vi "Data Format_old.vi"() -> (0 "title":string[](array[string]), 1 "title_beforedata":string[](array[string])=["Date", "Time", "Test_Time", "Station_Name", "Station_ID", "Variant", "Cavity_ID", "Operator_ID", "Serial_Number", "MES_DDM_SN", "Attempt_Time", "ETS_No", "MES", "SKU", "Plate_Diameter", "Overall_Result", "Error_Code", "Error_Description", "Run_Mode"], 3 "数组":string[][](array[string]))   [LabVIEW 2017]
panel:
  out "Table":string[][](array[string])
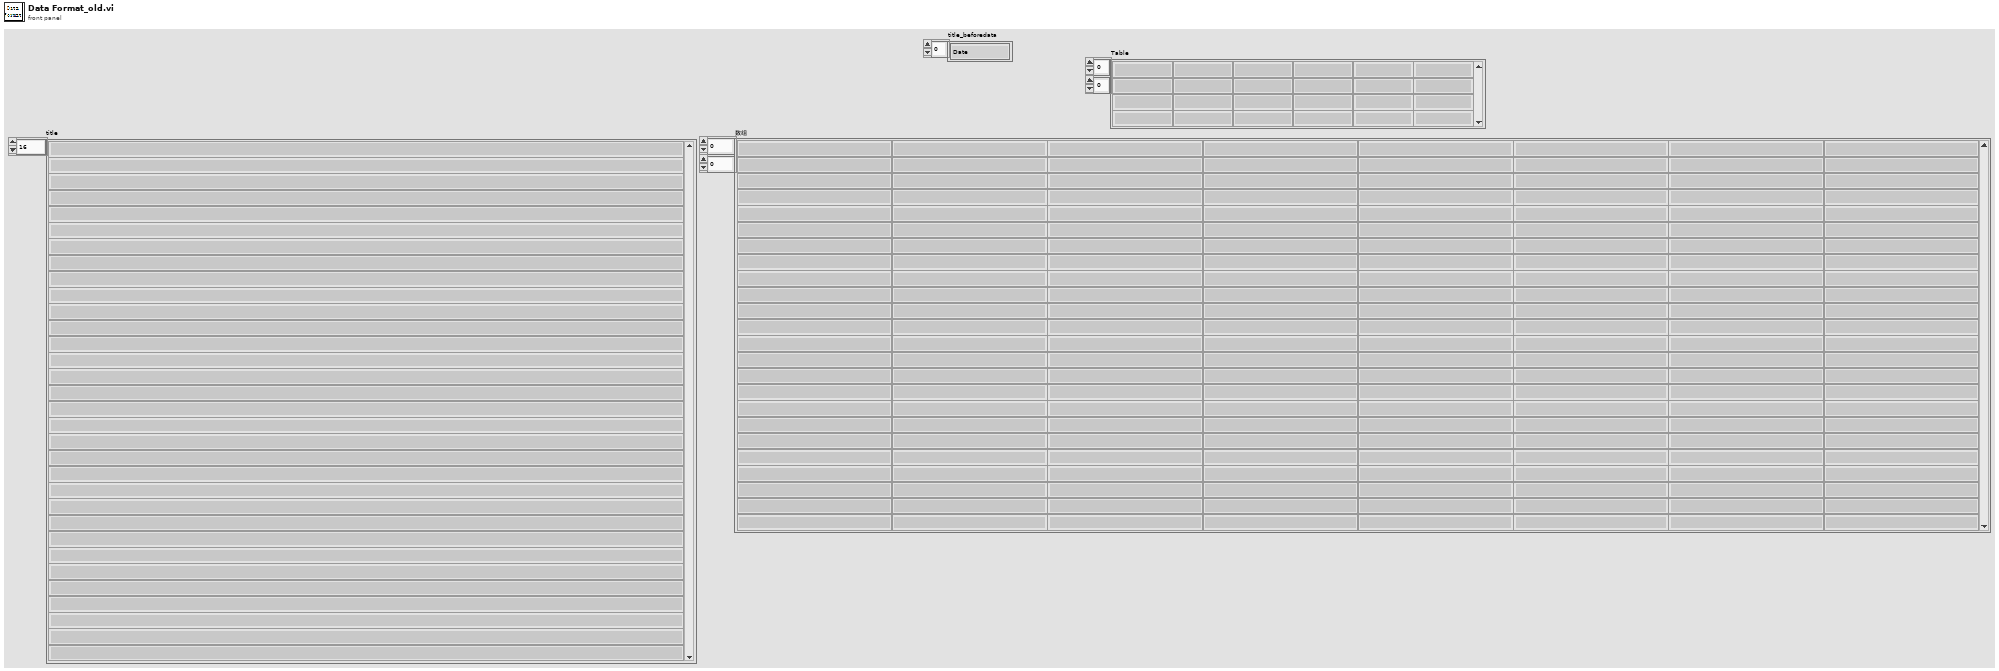
[diagram p1: front panel]
types:
  T1 = typedef "HD Config.ctl" = cluster{" PC":cluster{"PC Address":u8[], "PC Port":i32}, "FCO":cluster{"COM":refnum<visa-resource-name>, "Baudrate":u32}, "DC Power ":cluster{"COM":refnum<visa-resource-name>, "Baudrate":u32}, "PW3336":cluster{"COM":refnum<visa-resource-name>, "Baudrate":u32}, "Lefoo":cluster{"COM":refnum<visa-resource-name>, "Baudrate":u32}, "Tempt&Hum":cluster{"COM":refnum<visa-resource-name>, "Baudrate":u32}, "DIPC":cluster{"COM":refnum<visa-resource-name>}, "Daemon":cluster{"IP Address":string, "Port":u16, "Retry":u16}, "Motor":cluster{"COM":refnum<visa-resource-name>, "Baudrate":u32}, "Fail_resume_mode":bool, "GRR":bool}
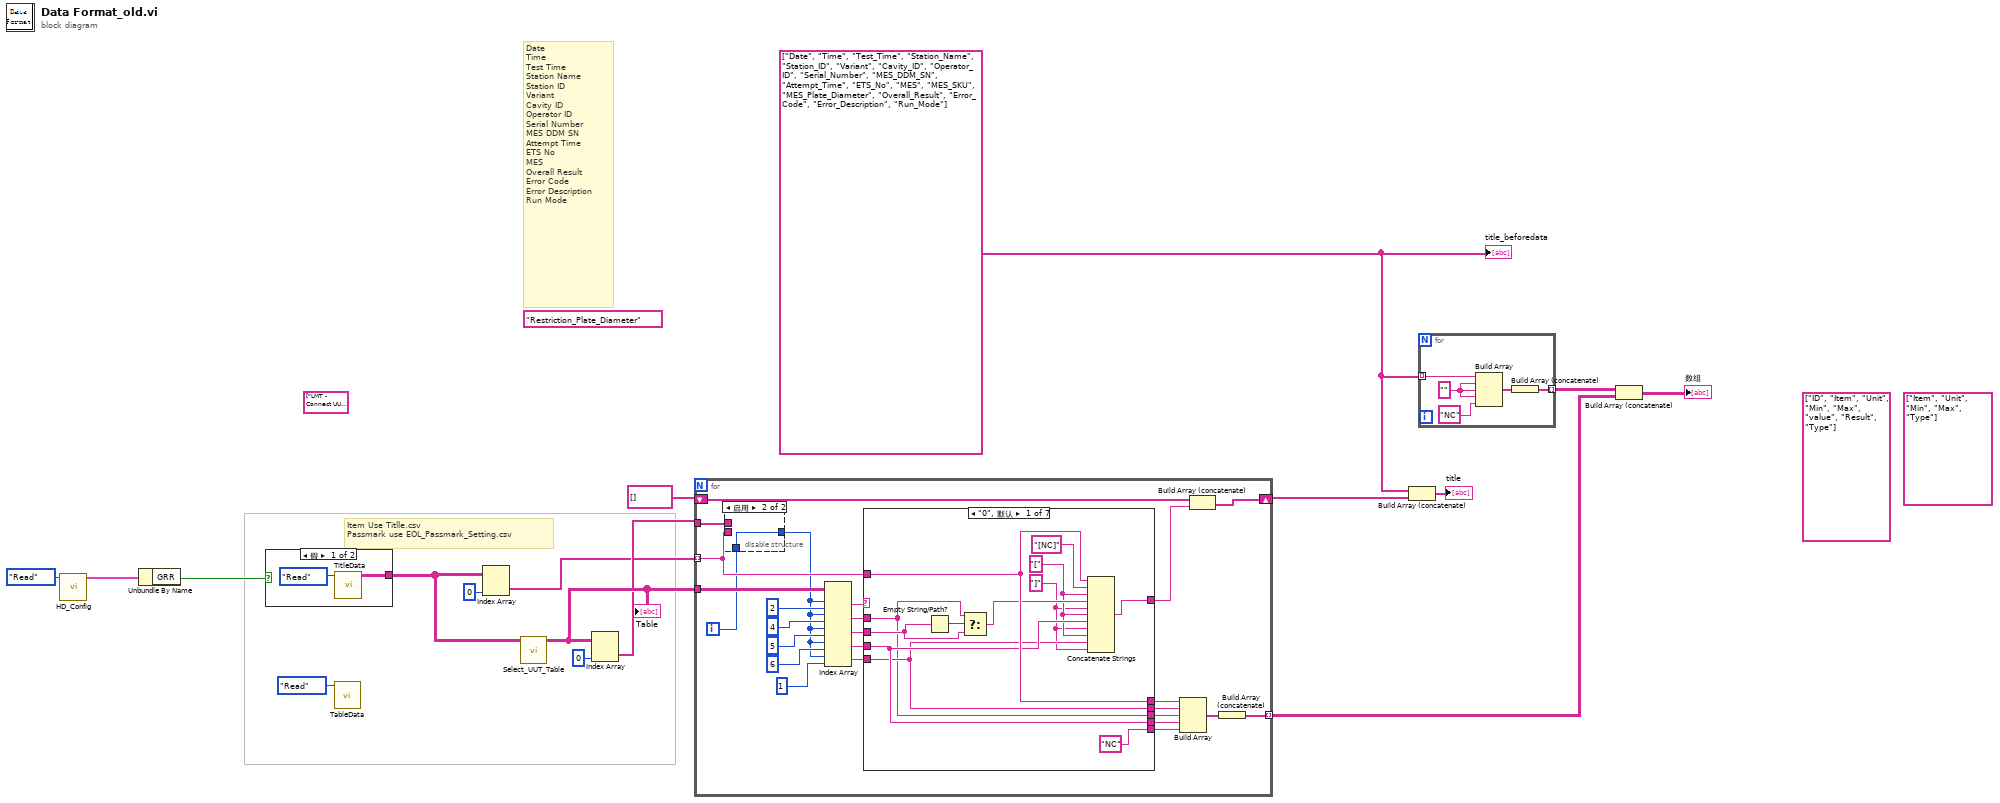
[diagram p0: block diagram]
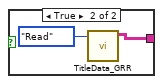
[diagram p2: hidden frame]
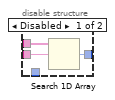
[diagram p3: hidden frame]
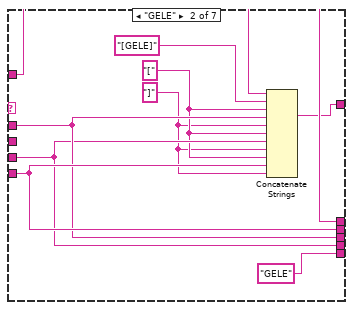
[diagram p4: hidden frame]
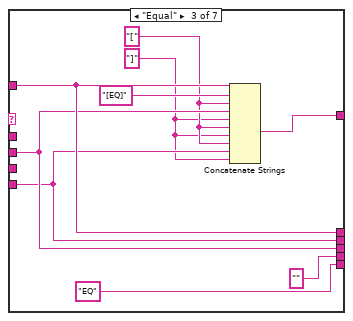
[diagram p5: hidden frame]
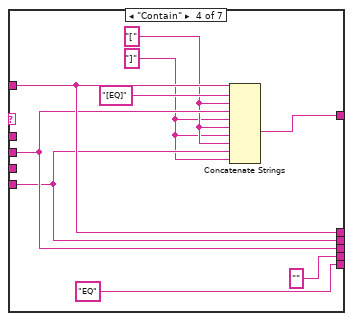
[diagram p6: hidden frame]
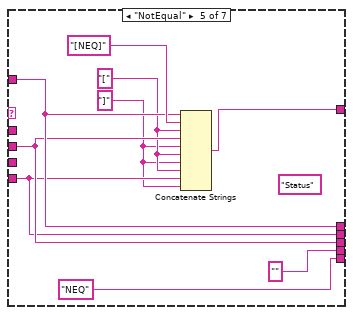
[diagram p7: hidden frame]
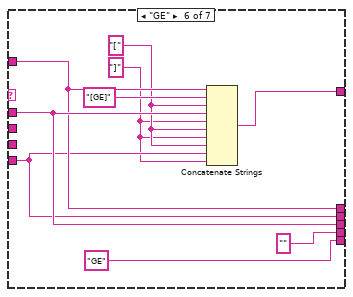
[diagram p8: hidden frame]
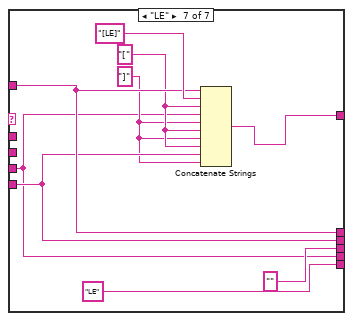
[diagram p9: hidden frame]
diagram:
  (unwired) "Restriction_Plate_Diameter"
  (unwired) string[] ["ID", "Item", "Unit", "Min", "Max", "value", "Result", "Type"] ("列首字符串[]")
  (unwired) string[] ["LMT - Connect UUT (con COM)", "LMT - Software Version (rrel)", "LMT - Write SKU file (wskuc)", "LMT - SKU file name", "LMT Connect UUT - Error Log", "5.3.2.1 Connect UUT DDM", "Connect UUT DDM - Error Log", "5.3.2.8 Read DDM EOL Timestamp", "5.3.2.8 Read DDM EOL Timestamp - Mode", "5.3.2.8 Read DDM EOL Timestamp - Timestamp", "5.3.2.8 Read DDM EOL Timestamp - Rig ID", "5.3.2.8 Read DDM EOL Timestamp - Passmark ID", "5.3.2.8 Read DDM EOL Timestamp - Passmark Rev", "Read DDM EOL Timestamp - Error Log", "5.3.2.2 Read DDM SW Version before flashing", "5.3.2.2 Software Version before flashing", "Read DDM SW Version before flashing - Error Log", "5.3.2.7 Read Hardware Serial", "Read Hardware Serial - Error Log", "Read DDM SN from UUT", "UUT DDM SN", "Compare Length", "Compare DDM SN with MES SN", "Check DDM SN - Error Log", "5.3.6.2.2 Backup File Data - CAL", "5.3.6.2.2 Backup Data Response - CAL", "5.3.2.3 Flash Firmware Version", "5.3.2.4 Wait Timeout", "5.3.2.5 Check SW Version", "5.3.2.5 Flashing firmware file name", "Flash Firmware Version - Error Log", "5.3.2a.1 Disconnect UUT", "Disconnect UUT - Error Log", "5.3.2a.3 Connect UUT UI", "Connect UUT UI - Error Log", "5.3.2a.4 Flash Firmware Version", "5.3.2a.4 Wait Timeout", "5.3.2a.4 Check SW Version", "5.3.2a.5 Flashing firmware file name", "Flash Firmware Version - Error Log", "5.3.2.6 Read DDM SW Version after flashing", "5.3.2.6 Check DDM SW Version after flashing", "Read DDM SW Version after flashing - Error Log", "5.3.2.10 Set SKU Config Status", "5.3.2.10 Set SKU Config", "5.3.2.10 Set SKU Config File Name", "Set SKU Config - Error Log", "5.3.2.10 Ready Status", "Ready Status - Error Log", "5.3.2.12 Set Device Mode to EOL", "5.3.2.12 DDM EOL mode", "Set Device Mode - Error Log", "5.3.4.34 Wait 1s", "5.3.2.13 DDM Parameter - Voltage", "5.3.2.13 DDM Parameter - Current", "5.3.2.13 DDM Parameter - Power", "5.3.2.13 DDM Parameter - Speed", "5.3.2.13 DDM Parameter - Pressure", "5.3.2.14 Tester Parameter - Voltage", "5.3.2.14 Tester Parameter - Current", "5.3.2.14 Tester Parameter - Power", "5.3.2.14 Tester Parameter - Ambient Pressure", "5.3.2.14 Tester Parameter - Ambient Temperature", "5.3.2.14 Tester Parameter - Pressure Box", "5.3.2.14 Tester Parameter - Reference Ambient Pressure", "5.3.2.15 Calculated Parameter - DDM Pressure Corrected", "5.3.2.15 Calculated Parameter - DDM Real Power", "5.3.2.15 Calculated Parameter - Delta V", "Get and Check Parameter - Error Log", "5.3.3.0 Read BEMF ambient temperature", "5.3.3.0 Calibration Result - eol_cold_bemf_temp", "Read BEMF ambient temperature - Error Log", "5.3.3.0 Set ambient temp to DDM", "5.3.3.0 DDM Ambient Temp", "Set ambient temp to DDM - Error Log", "5.3.4.2 Restriction Plate Diameter", "5.3.4.2 BEMF CAL - Put 13mm Restriction Plate", "Put Restriction Plate - Error Log", "5.3.3.1 Set - Calibrate BEMF both", "5.3.3.1 Get - Calibrate BEMF LSI", "5.3.3.2 Get - Calibration Result - eol_bemf_mp_cold_coef_a", "5.3.3.2 Get - Calibration Result - eol_bemf_mp_cold_coef_b", "5.3.3.2 Get - Calibration Result - eol_bemf_mp_cold_coef_c", "5.3.3.2 Get - Calibration Result - eol_bemf_lsi_cold_ref_coeffs", "5.3.3.2 Get - Calibration Result - eol_bemf_lsi_speed", "5.3.3.2 Get - Calibration Result - eol_bemf_lsi_integral_0", "5.3.3.2 Get - Calibration Result - eol_bemf_lsi_integral_1", "5.3.3.2 Get - Calibration Result - eol_bemf_lsi_integral_2", "5.3.3.2 Get - Calibration Result - eol_cold_bemf", "5.3.3.2 Get - Calibration Result - eol_cold_bemf_fisf", "Get - Calibrate BEMF LSI - Error Log", "5.3.3.3 Finalise Calibration", "5.3.3.4 Wait 1 sec", "Finalise Calibration - Error Log", "5.3.3.1 Get - Calibrate BEMF LSI", "5.3.3.2 Get - Calibration Result - eol_cold_bemf", "5.3.3.2 Get - Calibration Result - eol_cold_bemf_fisf", "5.3.3.2 Compare -Calibration Result - eol_cold_bemf", "5.3.3.2 Compare -Calibration Result - eol_cold_bemf_fisf", "Get & Compare - Calibrate BEMF LSI - Error Log", "5.3.3.3 Reset Power Tune", "5.3.3.4 Reset Power Tune Value", "Reset Power Tune - Error Log", "5.3.3.3 Reset BEMF FISF Calibration", "5.3.3.4 Reset BEMF FISF Calibration Value", "Reset BEMF FISF Calibration - Error Log", "5.3.4.2 ECO - Put 13mm Restriction Plate", "5.3.4.2 Restriction Plate Diameter", "Put Restriction Plate - Error Log", "5.3.4.5 ECO - Motor ON", "5.3.4.5 ECO - Motor ON Mode", "ECO - Motor ON - Error Log", "5.3.4.6 ECO - Motor Speed Stabilisation", "5.3.4.6 ECO - Stabilisation Time", "ECO - Motor Speed Stabilisation - Error Log", "5.3.4.7 ECO - DDM Parameter - Voltage", "5.3.4.7 ECO - DDM Parameter - Current", "5.3.4.7 ECO - DDM Parameter - Power", "5.3.4.7 ECO - DDM Parameter - Measured Power", "5.3.4.7 ECO - DDM Parameter - Speed", "5.3.4.7 ECO - DDM Parameter - Pressure", "5.3.4.7 ECO - DDM Parameter - lsi magnet temp", "5.3.4.7 ECO - DDM Parameter - fisf magnet temp", "5.3.4.7 ECO - DDM Parameter - iir magnet temp", "5.3.4.8 ECO - Tester Parameter - Voltage", "5.3.4.8 ECO - Tester Parameter - Current", "5.3.4.8 ECO - Tester Parameter - Power", "5.3.4.8 ECO - Tester Parameter - Ambient Pressure", "5.3.4.8 ECO - Tester Parameter - Ambient Temperature", "5.3.4.8 ECO - Tester Parameter - Ambient Humidity", "5.3.4.8 ECO - Tester Parameter - Pressure Box", "5.3.4.8 ECO - Tester Parameter - Reference Ambient Pressure", "5.3.4.9 ECO - Calculated Parameter - DDM Pressure Corrected", "5.3.4.9 ECO - Calculated Parameter - DDM Real Power", "5.3.4.9 ECO - Calculated Parameter - Delta V", "5.3.4.9 ECO - Calculated Parameter - Flowrate", "5.3.4.9 ECO - Calculated Parameter - Airwatt", "5.3.4.9 ECO - Formula", "ECO - Get and Check Parameter - Error Log", "PT ECO - Power Tune Mode Status", "PT ECO - Power Tune Set Delta Power Tune", "PT ECO - Power Tune Index", "PT ECO - Power Tune Delta_P", "PT ECO - Power Tune Motor ON Status", "PT ECO - Power Tune Motor ON Mode", "PT ECO - Power Tune Stabilisation Time Status", "PT ECO - Power Tune Stabilisation Delay Time", "PT ECO - DDM Parameter - Voltage", "PT ECO - DDM Parameter - Current", "PT ECO - DDM Parameter - Power", "PT ECO - DDM Parameter - Measured Power", "PT ECO - DDM Parameter - Speed", "PT ECO - DDM Parameter - Pressure", "PT ECO - DDM Parameter - lsi magnet temp", "PT ECO - DDM Parameter - fisf magnet temp", "PT ECO - DDM Parameter - iir magnet temp", "PT ECO - Tester Parameter - Voltage", "PT ECO - Tester Parameter - Current", "PT ECO - Tester Parameter - Power", "PT ECO - Tester Parameter - Ambient Pressure", "PT ECO - Tester Parameter - Ambient Temperature", "PT ECO - Tester Parameter - Ambient Humidity", "PT ECO - Tester Parameter - Pressure Box", "PT ECO - Tester Parameter - Reference Ambient Pressure", "PT ECO - Calculated Parameter - DDM Pressure Corrected", "PT ECO - Calculated Parameter - DDM Real Power", "PT ECO - Calculated Parameter - Delta V", "PT ECO - Calculated Parameter - Flowrate", "PT ECO - Calculated Parameter - Airwatt", "PT ECO - Formula", "PT ECO - Get and Check Parameter - Error Log", "5.3.4.2 BOOST - Put 13mm Restriction Plate", "5.3.4.2 Restriction Plate Diameter", "Put Restriction Plate - Error Log", "5.3.4.5 BOOST - Motor ON", "5.3.4.5 BOOST - Motor ON Mode", "BOOST - Motor ON - Error Log", "5.3.4.6 BOOST - Motor Speed Stabilisation", "5.3.4.6 BOOST - Stabilisation Time", "5.3.4.7 BOOST - DDM Parameter - Voltage", "5.3.4.7 BOOST - DDM Parameter - Current", "5.3.4.7 BOOST - DDM Parameter - Power", "5.3.4.7 BOOST - DDM Parameter - Measured Power", "5.3.4.7 BOOST - DDM Parameter - Speed", "5.3.4.7 BOOST - DDM Parameter - Pressure", "5.3.4.7 BOOST - DDM Parameter - lsi magnet temp", "5.3.4.7 BOOST - DDM Parameter - fisf magnet temp", "5.3.4.7 BOOST - DDM Parameter - iir magnet temp", "5.3.4.8 BOOST - Tester Parameter - Voltage", "5.3.4.8 BOOST - Tester Parameter - Current", "5.3.4.8 BOOST - Tester Parameter - Power", "5.3.4.8 BOOST - Tester Parameter - Ambient Pressure", "5.3.4.8 BOOST - Tester Parameter - Ambient Temperature", "5.3.4.8 BOOST - Tester Parameter - Ambient Humidity", "5.3.4.8 BOOST - Tester Parameter - Pressure Box", "5.3.4.8 BOOST - Tester Parameter - Reference Ambient Pressure", "5.3.4.9 BOOST - Calculated Parameter - DDM Pressure Corrected", "5.3.4.9 BOOST - Calculated Parameter - DDM Real Power", "5.3.4.9 BOOST - Calculated Parameter - Delta V", "5.3.4.9 BOOST - Calculated Parameter - Flowrate", "5.3.4.9 BOOST - Calculated Parameter - Airwatt", "5.3.4.9 BOOST - Formula", "BOOST - Get and Check Parameter - Error Log", "5.3.4.9 BOOST - Check air muscle presence", "5.3.4.9 BOOST - Check air muscle presence Vaule", "BOOST - Check air muscle presence - Error Log", "5.3.4.9 BOOST - Air Muscle Turn Off Status", "5.3.4.9 BOOST - Air Muscle Control", "5.3.3.10 BOOST - Air Muscle Stabilisation Time Status", "5.3.3.10 BOOST - Air Muscle Stabilisation Delay Time", "5.3.4.9 BOOST - Air Muscle Calculated Parameter - Airwatt B", "5.3.4.9 BOOST - Air Muscle Formula", "5.3.4.9 BOOST - Air Muscle Calculate Airwatt Delta", "BOOST - Air Muscle Check - Error Log", "PT BOOST - Power Tune Mode Status", "PT BOOST - Power Tune Set Delta Power Tune", "PT BOOST - Power Tune Index", "PT BOOST - Power Tune Delta_P", "PT BOOST - Power Tune Motor ON Status", "PT BOOST - Power Tune Motor ON Mode", "PT BOOST - Power Tune Stabilisation Time Status", "PT BOOST - Power Tune Stabilisation Delay Time", "PT BOOST - DDM Parameter - Voltage", "PT BOOST - DDM Parameter - Current", "PT BOOST - DDM Parameter - Power", "PT BOOST - DDM Parameter - Measured Power", "PT BOOST - DDM Parameter - Speed", "PT BOOST - DDM Parameter - Pressure", "PT BOOST - DDM Parameter - lsi magnet temp", "PT BOOST - DDM Parameter - fisf magnet temp", "PT BOOST - DDM Parameter - iir magnet temp", "PT BOOST - Tester Parameter - Voltage", "PT BOOST - Tester Parameter - Current", "PT BOOST - Tester Parameter - Power", "PT BOOST - Tester Parameter - Ambient Pressure", "PT BOOST - Tester Parameter - Ambient Temperature", "PT BOOST - Tester Parameter - Ambient Humidity", "PT BOOST - Tester Parameter - Pressure Box", "PT BOOST - Tester Parameter - Reference Ambient Pressure", "PT BOOST - Calculated Parameter - DDM Pressure Corrected", "PT BOOST - Calculated Parameter - DDM Real Power", "PT BOOST - Calculated Parameter - Delta V", "PT BOOST - Calculated Parameter - Flowrate", "PT BOOST - Calculated Parameter - Airwatt", "PT BOOST - Formula", "PT BOOST - Get and Check Parameter - Error Log", "5.3.4.34 Motor OFF", "5.3.4.34 Motor Power", "Motor OFF - Error Log", "5.3.4.34 Wait 1s", "5.3.4.35 Finalise Calibration", "Finalise Calibration - Error Log", "5.3.4.34 ECO - Get AW Calibration Status", "5.3.4.34 ECO - Get AW Calibration value", "5.3.4.34 ECO - Overall Status", "ECO - Get AW Calibration - Error Log", "5.3.4.34 BOOST - Get AW Calibration Status", "5.3.4.34 BOOST - Get AW Calibration value", "5.3.4.34 BOOST - Overall Status", "BOOST - Get AW Calibration - Error Log", "5.3.4.2 MAX - Put 13mm Restriction Plate", "5.3.4.2 Restriction Plate Diameter", "Put Restriction Plate - Error Log", "5.3.4.5 MAX - Motor ON", "5.3.4.5 MAX - Motor ON Mode", "MAX - Motor ON - Error Log", "5.3.4.6 MAX - Motor Speed Stabilisation", "5.3.4.6 MAX - Stabilisation Time", "MAX - Motor Speed Stabilisation - Error Log", "5.3.4.6 Get Average Delta Tmag Status", "5.3.4.6 Get Average Delta Tmag (LSIdelta_FISFdelta_LSItmag_FISFtmag_IIRtmag)", "5.3.4.6 Get Average Delta Tmag LSI", "5.3.4.6 Get Average Delta Tmag FISF", "Get Average Delta Tmag - Error Log", "5.3.4.7 MAX - DDM Parameter - Voltage", "5.3.4.7 MAX - DDM Parameter - Current", "5.3.4.7 MAX - DDM Parameter - Power", "5.3.4.7 MAX - DDM Parameter - Measured Power", "5.3.4.7 MAX - DDM Parameter - Speed", "5.3.4.7 MAX - DDM Parameter - Pressure", "5.3.4.8 MAX - Tester Parameter - Voltage", "5.3.4.8 MAX - Tester Parameter - Current", "5.3.4.8 MAX - Tester Parameter - Power", "5.3.4.8 MAX - Tester Parameter - Ambient Pressure", "5.3.4.8 MAX - Tester Parameter - Ambient Temperature", "5.3.4.8 MAX - Tester Parameter - Ambient Humidity", "5.3.4.8 MAX - Tester Parameter - Pressure Box", "5.3.4.8 MAX - Tester Parameter - Reference Ambient Pressure", "5.3.4.9 MAX - Calculated Parameter - DDM Pressure Corrected", "5.3.4.9 MAX - Calculated Parameter - DDM Real Power", "5.3.4.9 MAX - Calculated Parameter - Delta V", "5.3.4.9 MAX - Calculated Parameter - Flowrate", "5.3.4.9 MAX - Calculated Parameter - Airwatt", "5.3.4.9 MAX - Formula", "MAX - Get and Check Parameter - Error Log", "5.3.3.10 MAX - FISF - Check Average Delta Tmag", "5.3.3.10 MAX - FISF - Check Average Delta Tmag Status", "5.3.3.10 MAX - FISF - BEMF Finetune Result", "BEMF Finetune - Error Log", "MAX tune - Check Airwatts Status", "Calculate Delta Airwatts - MAX tune - Calculate Delta Airwatts", "Calculate Delta Airwatts a - MAX tune - ddm_real_power_a", "Calculate Delta Airwatts b - MAX tune - ddm_real_power_b", "Calculate Delta Airwatts c - MAX tune - Target AW", "Calculate Delta Airwatts d - MAX tune - AW tune extra", "Calculate Delta Airwatts e - MAX tune - Latest AW", "Calculate Delta Airwatts f - MAX tune - correction_factor", "Calculate Delta Airwatts g - MAX tune - P extra", "Calculate Delta Airwatts h - MAX tune - constant power table index", "Calculate Delta Airwatts - MAX tune - Delta P1", "Set AW Tune - MAX tune - Daemon Status", "Set AW Tune - MAX tune - Delta P1 in mW", "Set AW Tune - MAX tune - constant power table index", "Set AW Tune - MAX tune - Drive Mode", "Set AW Tune - MAX tune - Result Airwatt Tune", "5.3.4.5 MAX tune - Motor ON", "5.3.4.5 MAX tune - Motor ON Mode", "5.3.4.6 MAX tune - Motor Speed Stabilisation", "5.3.4.6 MAX tune - Stabilisation Time", "5.3.4.7 MAX tune - DDM Parameter - Voltage", "5.3.4.7 MAX tune - DDM Parameter - Current", "5.3.4.7 MAX tune - DDM Parameter - Power", "5.3.4.7 MAX tune - DDM Parameter - Measured Power", "5.3.4.7 MAX tune - DDM Parameter - Speed", "5.3.4.7 MAX tune - DDM Parameter - Pressure", "5.3.4.7 MAX tune - DDM Parameter - lsi magnet temp", "5.3.4.7 MAX tune - DDM Parameter - fisf magnet temp", "5.3.4.7 MAX tune - DDM Parameter - iir magnet temp", "5.3.4.8 MAX tune - Tester Parameter - Voltage", "5.3.4.8 MAX tune - Tester Parameter - Current", "5.3.4.8 MAX tune - Tester Parameter - Power", "5.3.4.8 MAX tune - Tester Parameter - Ambient Pressure", "5.3.4.8 MAX tune - Tester Parameter - Ambient Temperature", "5.3.4.8 MAX tune - Tester Parameter - Ambient Humidity", "5.3.4.8 MAX tune - Tester Parameter - Pressure Box", "5.3.4.8 MAX tune - Tester Parameter - Reference Ambient Pressure", "5.3.4.9 MAX tune - Calculated Parameter - DDM Pressure Corrected", "5.3.4.9 MAX tune - Calculated Parameter - DDM Real Power", "5.3.4.9 MAX tune - Calculated Parameter - Delta V", "5.3.4.9 MAX tune - Calculated Parameter - Flowrate", "5.3.4.9 MAX tune - Calculated Parameter - Airwatt", "5.3.4.9 MAX tune - Formula", "MAX tune - Get and Check Parameter - Error Log", "MAX finetune - Check Airwatts Status", "Calculate Delta Airwatts - MAX finetune - Calculate Delta Airwatts", "Calculate Delta Airwatts a - MAX finetune - ddm_real_power_a", "Calculate Delta Airwatts b - MAX finetune - ddm_real_power_b", "Calculate Delta Airwatts c - MAX finetune - Target AW", "Calculate Delta Airwatts d - MAX finetune - AW tune extra", "Calculate Delta Airwatts e - MAX finetune - Latest AW", "Calculate Delta Airwatts f - MAX finetune - correction_factor", "Calculate Delta Airwatts g - MAX finetune - P extra", "Calculate Delta Airwatts h - MAX finetune - constant power table index", "Calculate Delta Airwatts - MAX finetune - Delta P2", "Set AW Tune - MAX finetune - Daemon Status", "Set AW Tune - MAX finetune - Delta P2 in mW", "Set AW Tune - MAX finetune - constant power table index", "Set AW Tune - MAX finetune - Drive Mode", "Set AW Tune - MAX finetune - Result Airwatt Finetune", "5.3.4.5 MAX finetune - Motor ON", "5.3.4.5 MAX finetune - Motor ON Mode", "5.3.4.6 MAX finetune - Motor Speed Stabilisation", "5.3.4.6 MAX finetune - Stabilisation Time", "5.3.4.7 MAX finetune - DDM Parameter - Voltage", "5.3.4.7 MAX finetune - DDM Parameter - Current", "5.3.4.7 MAX finetune - DDM Parameter - Power", "5.3.4.7 MAX finetune - DDM Parameter - Measured Power", "5.3.4.7 MAX finetune - DDM Parameter - Speed", "5.3.4.7 MAX finetune - DDM Parameter - Pressure", "5.3.4.7 MAX finetune - DDM Parameter - lsi magnet temp", "5.3.4.7 MAX finetune - DDM Parameter - fisf magnet temp", "5.3.4.7 MAX finetune - DDM Parameter - iir magnet temp", "5.3.4.8 MAX finetune - Tester Parameter - Voltage", "5.3.4.8 MAX finetune - Tester Parameter - Current", "5.3.4.8 MAX finetune - Tester Parameter - Power", "5.3.4.8 MAX finetune - Tester Parameter - Ambient Pressure", "5.3.4.8 MAX finetune - Tester Parameter - Ambient Temperature", "5.3.4.8 MAX finetune - Tester Parameter - Ambient Humidity", "5.3.4.8 MAX finetune - Tester Parameter - Pressure Box", "5.3.4.8 MAX finetune - Tester Parameter - Reference Ambient Pressure", "5.3.4.9 MAX finetune - Calculated Parameter - DDM Pressure Corrected", "5.3.4.9 MAX finetune - Calculated Parameter - DDM Real Power", "5.3.4.9 MAX finetune - Calculated Parameter - Delta V", "5.3.4.9 MAX finetune - Calculated Parameter - Flowrate", "5.3.4.9 MAX finetune - Calculated Parameter - Airwatt", "5.3.4.9 MAX finetune - Formula", "MAX finetune - Get and Check Parameter - Error Log", "5.3.3.10 Check Derate Status", "5.3.3.10 Check Derate Result", "Check Derate Status - Get and Check Parameter - Error Log", "5.3.4.6 Get Delta Tmag After Tuned Status", "5.3.4.6 Delta Tmag FISF", "5.3.4.6 FISF Tmag", "5.3.4.6 IIR Tmag", "Get Delta Tmag After Tuned - Error Log", "5.3.3.10 Get Hot BEMF Status", "5.3.3.10 Get Hot BEMF Result", "Get Hot BEMF Status - Get and Check Parameter - Error Log", "5.3.4.34 Motor OFF", "5.3.4.34 Motor Power", "Motor OFF - Error Log", "5.3.4.34 Wait 1s", "Wait - Error Log", "5.3.3.10 Get DDM Pressure Status", "5.3.3.10 DDM Pressure", "5.3.3.10 Tester Ambient Pressure", "5.3.3.10 Calculate delta Pressure", "Get DDM Pressure Status - Get and Check Parameter - Error Log", "5.3.4.35 Finalise Calibration", "5.3.4.36 Wait 1 sec", "Finalise Calibration - Error Log", "5.3.3.0 Get Cold BEMF Status", "5.3.3.0 Get Cold BEMF - eol_cold_bemf_fisf", "5.3.3.0 Calculate & Check Delta BEMF", "Get Cold BEMF fisf - Error Log", "5.3.4.34 Get AW Calibration Status", "5.3.4.34 Delta P Airwatts Value", "5.3.4.34 Get Airwatts Tune Index 2", "5.3.4.34 Compare Result", "Get AW Calibration - Error Log", "5.3.3.0 Read DDM ambient temperature", "5.3.3.0 Calibration Result - eol_cold_bemf_temp", "Read BEMF ambient temperature - Error Log", "5.3.3.0 Set ambient temp to DDM", "5.3.3.0 DDM Ambient Temp", "Set ambient temp to DDM - Error Log", "5.3.5.1 Reset Task Detect - LL", "5.3.5.1 Reset Task Detect - HL", "5.3.5.1 Reset Task Detect - LH", "5.3.5.1 Reset Task Detect - HH", "5.3.5.1 Reset eol inlet blockage", "5.3.5.2 LL - Put 30mm Restriction Plate", "5.3.5.2 Restriction Plate Diameter", "Put Restriction Plate - Error Log", "5.3.5.4 LL - A2 mode Motor ON", "5.3.5.4 LL - A2 mode Motor Power", "LL -A2 mode Motor ON - Error Log", "5.3.5.5 LL - Motor Speed Stabilisation", "5.3.5.5 LL - Stabilisation Time", "LL - Motor Speed Stabilisation - Error Log", "5.3.5.6 LL - DDM Parameter - Voltage", "5.3.5.6 LL - DDM Parameter - Current", "5.3.5.6 LL - DDM Parameter - Power", "5.3.5.6 LL - DDM Parameter - Measured Power", "5.3.5.6 LL - DDM Parameter - Speed", "5.3.5.6 LL - DDM Parameter - Pressure", "5.3.5.7 LL - Tester Parameter - Voltage", "5.3.5.7 LL - Tester Parameter - Current", "5.3.5.7 LL - Tester Parameter - Power", "5.3.5.7 LL - DDM Real Power", "5.3.5.7 LL - Get and Check Parameter - Error Log", "5.3.5.8 LL - Calibrate Task Detect LL", "5.3.5.8 LL - Set Calibrate Task Detect LL", "5.3.5.8 LL - Calibrate Task Detect - Error Log", "5.3.5.4 HL - BOOST mode Motor ON", "5.3.5.4 HL - BOOST mode Motor Power", "HL - BOOST mode Motor ON - Error Log", "5.3.5.5 HL - Motor Speed Stabilisation", "5.3.5.5 HL - Stabilisation Time", "HL - Motor Speed Stabilisation - Error Log", "5.3.5.6 HL - DDM Parameter - Voltage", "5.3.5.6 HL - DDM Parameter - Current", "5.3.5.6 HL - DDM Parameter - Power", "5.3.5.6 HL - DDM Parameter - Measured Power", "5.3.5.6 HL - DDM Parameter - Speed", "5.3.5.6 HL - DDM Parameter - Pressure", "5.3.5.7 HL - Tester Parameter - Voltage", "5.3.5.7 HL - Tester Parameter - Current", "5.3.5.7 HL - Tester Parameter - Power", "5.3.5.7 HL - DDM Real Power", "5.3.5.7 HL - Get and Check Parameter - Error Log", "5.3.5.8 HL - Calibrate Task Detect HL", "5.3.5.8 HL - Set Calibrate Task Detect HL", "5.3.5.8 HL - Calibrate Task Detect - Error Log", "5.3.5.15 Motor OFF", "5.3.5.15 Motor Power", "Motor OFF - Error Log", "5.3.5.15 Wait 1s", "Wait - Error Log", "5.3.5.2 LH - Put 16mm Restriction Plate", "5.3.5.2 Restriction Plate Diameter", "Put Restriction Plate - Error Log", "5.3.5.4 LH -A2 mode Motor ON", "5.3.5.4 LH - A2 mode Motor Power", "LH - A2 mode Motor ON - Error Log", "5.3.5.5 LH - Motor Speed Stabilisation", "5.3.5.5 LH - Stabilisation Time", "LH - Motor Speed Stabilisation - Error Log", "5.3.5.6 LH - DDM Parameter - Voltage", "5.3.5.6 LH - DDM Parameter - Current", "5.3.5.6 LH - DDM Parameter - Power", "5.3.5.6 LH - DDM Parameter - Measured Power", "5.3.5.6 LH - DDM Parameter - Speed", "5.3.5.6 LH - DDM Parameter - Pressure", "5.3.5.7 LH - Tester Parameter - Voltage", "5.3.5.7 LH - Tester Parameter - Current", "5.3.5.7 LH - Tester Parameter - Power", "5.3.5.7 LH - DDM Real Power", "5.3.5.7 LH - Get and Check Parameter - Error Log", "5.3.5.8 LH - Calibrate Task Detect LH", "5.3.5.8 LH - Set Calibrate Task Detect LH", "5.3.5.8 LH - Calibrate Task Detect - Error Log", "5.3.5.4 HH - BOOST mode Motor ON", "5.3.5.4 HH - BOOST mode Motor Power", "HH - BOOST mode Motor ON - Error Log", "5.3.5.5 HH - Motor Speed Stabilisation", "5.3.5.5 HH - Stabilisation Time", "HH - Motor Speed Stabilisation - Error Log", "5.3.5.6 HH - DDM Parameter - Voltage", "5.3.5.6 HH - DDM Parameter - Current", "5.3.5.6 HH - DDM Parameter - Power", "5.3.5.6 HH - DDM Parameter - Measured Power", "5.3.5.6 HH - DDM Parameter - Speed", "5.3.5.6 HH - DDM Parameter - Pressure", "5.3.5.7 HH - Tester Parameter - Voltage", "5.3.5.7 HH - Tester Parameter - Current", "5.3.5.7 HH - Tester Parameter - Power", "5.3.5.7 HH - DDM Real Power", "5.3.5.7 HH - Get and Check Parameter - Error Log", "5.3.5.8 HH - Calibrate Task Detect HH", "5.3.5.8 HH - Set Calibrate Task Detect HH", "5.3.5.8 HH - Calibrate Task Detect - Error Log", "5.3.5.29 Wait 1s", "Wait - Error Log", "Inlet Blockage Calibration - Motor ON", "Inlet Blockage Calibration - Motor Power", "Inlet Blockage Calibration - Motor ON - Error Log", "Inlet Blockage Calibration - Motor Speed Stabilisation", "Inlet Blockage Calibration - Stabilisation Time", "Inlet Blockage Calibration - Motor Speed Stabilisation - Error Log", "Inlet Blockage Calibration - DDM Parameter - Voltage", "Inlet Blockage Calibration - DDM Parameter - Current", "Inlet Blockage Calibration - DDM Parameter - Power", "Inlet Blockage Calibration - DDM Parameter - Measured Power", "Inlet Blockage Calibration - DDM Parameter - Speed", "Inlet Blockage Calibration - DDM Parameter - Pressure", "Inlet Blockage Calibration - DDM Parameter - lsi magnet temp", "Inlet Blockage Calibration - DDM Parameter - fisf magnet temp", "Inlet Blockage Calibration - DDM Parameter - iir magnet temp", "Inlet Blockage Calibration - Tester Parameter - Voltage", "Inlet Blockage Calibration - Tester Parameter - Current", "Inlet Blockage Calibration - Tester Parameter - Power", "Inlet Blockage Calibration - DDM Real Power", "Inlet Blockage Calibration - Get and Check Parameter - Error Log", "5.3.5.30 Set Calibrate Inlet Blockage", "5.3.5.30 Calibrate Inlet Blockage Value", "5.3.5.31 Calibrate Inlet Blockage - Wait 1s", "Calibrate Inlet Blockage - Error Log", "5.3.5.15 Motor OFF", "5.3.5.15 Motor Power", "Motor OFF - Error Log", "5.3.5.32 Wait 1s", "Wait - Error Log", "5.3.5.35 Get Calibration Inlet Blockage", "5.3.5.35 Calibration Inlet Blockage", "Get Calibration Inlet Blockage - Error Log", "5.3.3.0 Set ambient temp to DDM", "5.3.3.0 DDM Ambient Temp", "Set ambient temp to DDM - Error Log", "5.3.5.33 Finalise Calibration", "5.3.5.34 Wait 1 sec", "Finalise Calibration - Error Log", "5.3.5.35 Get Task Detect LL", "5.3.5.35 Get Task Detect HL", "5.3.5.35 Get Task Detect LH", "5.3.5.35 Get Task Detect HH", "Get Task Detect - Error Log", "5.3.5.35 Get Calibration Inlet Blockage", "5.3.5.35 Calibration Inlet Blockage", "5.3.5.35 Calibration eol cold bemf temp", "5.3.5.35 Compare Task Detect LL", "5.3.5.35 Compare Task Detect HL", "5.3.5.35 Compare Task Detect LH", "5.3.5.35 Compare Task Detect HH", "5.3.5.35 Compare Calibration Inlet Blockage", "5.3.5.35 Compare Calibration eol cold bemf temp", "Compare Task Detect Inlet Blockage - Error Log", "5.3.6.1.2 GOOD UNIT - Clear EEPROM Error Log", "GOOD UNIT - Clear EEPROM Error Log - Error Log", "5.3.6.1.3 GOOD UNIT - Write Product Timestamp", "5.3.6.1.3 GOOD UNIT - Write Product Timestamp - Mode", "5.3.6.1.3 GOOD UNIT - Write Product Timestamp - Timestamp", "5.3.6.1.3 GOOD UNIT - Write Product Timestamp - Rig ID", "5.3.6.1.3 GOOD UNIT - Write Product Timestamp - Passmark ID", "5.3.6.1.3 GOOD UNIT - Write Product Timestamp - Passmark Rev", "GOOD UNIT - Write Product Timestamp - Error Log", "5.3.2.12 GOOD UNIT - Set Device Mode to PROD", "5.3.2.12 GOOD UNIT - DDM PROD mode", "GOOD UNIT - Set Device Mode - Error Log", "5.3.6.1.6 GOOD UNIT - Wait 1s Delay", "GOOD UNIT - Delay - Error Log", "5.3.2.8 GOOD UNIT - Read DDM PROD Timestamp", "5.3.2.8 GOOD UNIT - Read DDM PROD Timestamp - Mode", "5.3.2.8 GOOD UNIT - Read DDM PROD Timestamp - Timestamp", "5.3.2.8 GOOD UNIT - Read DDM PROD Timestamp - Rig ID", "5.3.2.8 GOOD UNIT - Read DDM PROD Timestamp - Passmark ID", "5.3.2.8 GOOD UNIT - Read DDM PROD Timestamp - Passmark Rev", "5.3.2.8 Compare - Read DDM PROD Timestamp", "5.3.2.8 Compare - Read DDM PROD Timestamp - Mode", "5.3.2.8 Compare - Read DDM PROD Timestamp - Timestamp", "5.3.2.8 Compare - Read DDM PROD Timestamp - Rig ID", "5.3.2.8 Compare - Read DDM PROD Timestamp - Passmark ID", "5.3.2.8 Compare - Read DDM PROD Timestamp - Passmark Rev", "GOOD UNIT - Read DDM PROD Timestamp - Error Log", "5.3.6.1.7 GOOD UNIT - Backup File Data", "5.3.6.1.7 GOOD UNIT - Backup File Data  - Error Log", "5.3.2.7 GOOD UNIT - Check Security Bit", "GOOD UNIT - Check Security Bit - Error Log", "5.3.6.1.8 GOOD UNIT - Set Calibration Lock", "GOOD UNIT - Set Calibration Lock - Error Log", "5.3.6.1.9 GOOD UNIT - Disconnect UUT", "GOOD UNIT - Disconnect UUT - Error Log", "5.3.6.2.2 NG UNIT - Read NVM Error", "NG UNIT - Read NVM Error - Error Log", "5.3.2.12 NG UNIT - DDM FCT mode", "5.3.2.12 NG UNIT - DDM FCT mode", "NG UNIT - Set Device Mode - Error Log", "5.3.6.2.2 NG UNIT - Backup File Data - CAL", "5.3.6.2.2 NG UNIT - Backup File Data - ERROR", "5.3.6.2.2 NG UNIT - Backup File Data - USAGE", "NG UNIT - Backup File Data - Error Log", "5.3.6.2.4 NG UNIT - Disconnect UUT", "NG UNIT - Disconnect UUT - Error Log"] ("数组 2")
  (unwired) string[] ["Item", "Unit", "Min", "Max", "Type"] ("列首字符串[]")
  w2 = string[] ["Date", "Time", "Test_Time", "Station_Name", "Station_ID", "Variant", "Cavity_ID", "Operator_ID", "Serial_Number", "MES_DDM_SN", "Attempt_Time", "ETS_No", "MES", "MES_SKU", "MES_Plate_Diameter", "Overall_Result", "Error_Code", "Error_Description", "Run_Mode"]
  # "Date\nTime\nTest Time\nStation Name\nStation ID\nVariant\nCavity ID\nOperator ID\nSerial Number\nMES DDM SN\nAttempt Time\nETS No\nMES\nOverall Result\nError Code\nError Description\nRun Mode"
  # "Item Use Titlle.csv\nPassmark use EOL_Passmark_Setting.csv"
  n1 = call "HD_Config.vi"("Step"=enum16{"Initial", "Write", "Read"}."Read") -> ("HD Config out"=w6:T1)  [unwired: 9 in, 1 out]
  n2 = Unbundle By Name(w6) -> ("GRR"=w5:bool)
  n3 = case shown="假" w5 {
    tunnel: [w18 w20] -> w9
    frame False {
      n4 = call "TitleData.vi"("Step"=enum16{"Initial", "Write", "Read"}."Read") -> ("Tabledata Out"=w18:string[][])  [unwired: 9 in, 1 out]
    }
    frame True {
      n5 = call "TitleData_GRR.vi"("Step"=enum16{"Initial", "Write", "Read"}."Read") -> ("Tabledata Out"=w20:string[][])  [unwired: 9 in, 1 out]
    }
  }
  n6 = call "TableData.vi"("Step"=enum16{"Initial", "Write", "Read"}."Read") -> ()  [unwired: 9 in, 2 out]
  n7 = Index Array "Index Array"(array=w9, index (col)=0 ("禁用的索引 (列)")) -> (element=w10:string[])  [unwired: 1 in]
  n8 = call "Select_UUT_Table.vi"("all Table"=w9) -> ("Table"=w16:string[][])  [unwired: 9 in, 1 out]
  "Table" <- w16
  n9 = Index Array(array=w16, index (col)=0 ("禁用的索引 (列)")) -> (element=w14:string[])  [unwired: 1 in]
  n10 = for {
    tunnel: w10 -> [w34] mode=indexing
    tunnel: w16 -> [w45]
    tunnel: w14 -> [w46]
    shift-right: [w35] -> w12
    shift-left: string[] [] -> [w36]
    tunnel: [w27] -> w3 mode=indexing
    i -> [w22]
    n11 = disable-structure shown="启用" {
      disable-tunnel: w46 -> [w49 _]
      disable-tunnel: w34 -> [w48 _]
      disable-tunnel: [w47 w50] -> w24
      disable-tunnel: w22 -> [_ w50]
      frame Disabled {
        n12 = Search 1D Array(1D array=w49, element=w48) -> (index of element=w47:i32)  [unwired: 1 in]
      }
      frame Enabled {
      }
    }
    n13 = Index Array(array=w45, index (row) #1=w24, index (col) #1=2 ("禁用的索引 (列)"), index (row) #2=w24, index (col) #2=4 ("禁用的索引 (列)"), index (row) #3=w24, index (col) #3=5 ("禁用的索引 (列)"), index (row) #4=w24, index (col) #4=6 ("禁用的索引 (列)"), index (row) #5=w24, index (col) #5=1 ("索引 (列)")) -> (element #1=w43:string, element #2=w39:string, element #3=w38:string, element #4=w37:string, element #5=w25:string)
    n14 = case shown="\"0\", 默认" w43 {
      tunnel: w39 -> [w54 w66 _ _ _ w106 _]
      tunnel: w38 -> [w55 _ w77 w86 w95 _ _]
      tunnel: w37 -> [w58 w65 _ _ _ _ w108]
      tunnel: [w59 w68 w75 w84 w93 w102 w112] -> w23
      tunnel: w34 -> [w61 w70 w79 w88 w97 w105 w115]
      tunnel: [w61 w70 w79 w88 w97 w105 w115] -> w33
      tunnel: [w54 w66 w77 w86 w95 w106 "" ("String")] -> w32
      tunnel: [w58 w65 "" ("String") "" ("String") "" ("String") "" ("String") w108] -> w31
      tunnel: ["NC" "GELE" "EQ" "EQ" "NEQ" "GE" "LE"] -> w30
      tunnel: [w57 w67 w74 w83 w91 w101 w111] -> w28
      tunnel: w25 -> [w57 w67 w74 w83 w91 w101 w111]
      frame "0", Default {
        w51 = "]" ("字符串")
        w52 = "[" ("字符串")
        n15 = Empty String/Path?(string/path=w55) -> (empty?=w56:bool)
        n16 = Select(t=w54, s=w56, f=w55) -> (s? t:f=w53:string)
        n17 = Concatenate Strings(w61, "[NC]", w52, w53, w51, w52, w58, w51, w52, w57, w51) -> (w59:string)
      }
      frame "GELE" {
        w63 = "]" ("字符串")
        w64 = "[" ("字符串")
        n18 = Concatenate Strings(w70, "[GELE]", w64, w66, w63, w64, w65, w63, w64, w67, w63) -> (w68:string)
      }
      frame "Equal" {
        w72 = "]" ("字符串")
        w73 = "[" ("字符串")
        n19 = Concatenate Strings(w79, "[EQ]", w73, w77, w72, w73, w72, w73, w74, w72) -> (w75:string)
      }
      frame "Contain" {
        w81 = "]" ("字符串")
        w82 = "[" ("字符串")
        n20 = Concatenate Strings(w88, "[EQ]", w82, w86, w81, w82, w81, w82, w83, w81) -> (w84:string)
      }
      frame "NotEqual" {
        (unwired) "Status" ("元素")
        w90 = "]" ("字符串")
        w92 = "[" ("字符串")
        n21 = Concatenate Strings(w97, "[NEQ]", w92, w95, w90, w92, w90, w92, w91, w90) -> (w93:string)
      }
      frame "GE" {
        w99 = "]" ("字符串")
        w100 = "[" ("字符串")
        n22 = Concatenate Strings(w105, "[GE]", w100, w106, w99, w100, w99, w100, w101, w99) -> (w102:string)
      }
      frame "LE" {
        w109 = "]" ("字符串")
        w110 = "[" ("字符串")
        n23 = Concatenate Strings(w115, "[LE]", w110, w108, w109, w110, w109, w110, w111, w109) -> (w112:string)
      }
    }
    n24 = Build Array ("创建数组")(w33, w28, w32, w31, w30) -> (w29:string[])
    n25 = Build Array (concatenate)(w36, w23) -> (w35:string[])
    n26 = Build Array (concatenate) ("创建数组")(w29) -> (w27:string[])
  }
  n27 = Build Array (concatenate)(w2, w12) -> (→"title":string[])
  n28 = for {
    tunnel: w2 -> [w118] mode=indexing
    tunnel: [w120] -> w4 mode=indexing
    w117 = ""
    n29 = Build Array(w118, w117, w117, w117, "NC") -> (w121:string[])
    n30 = Build Array (concatenate)(w121) -> (w120:string[])
  }
  n31 = Build Array (concatenate)(w4, w3) -> (→"数组":string[][])
  "title_beforedata" <- w2
